vi "PicoLog_DATA.vi"(3 "sampleInterval_ms":dbl, 4 "handle":i16, 5 "noOfChannels":i16) -> (0 "Sensor3":i32[](graph), 1 "Waveform Graph 3":dynamicdata(graph), 2 "handle":i16)   [LabVIEW 2014]
uses:
  picohrdl.dll
panel:
  out "Sensor3 2":dynamicdata(graph)
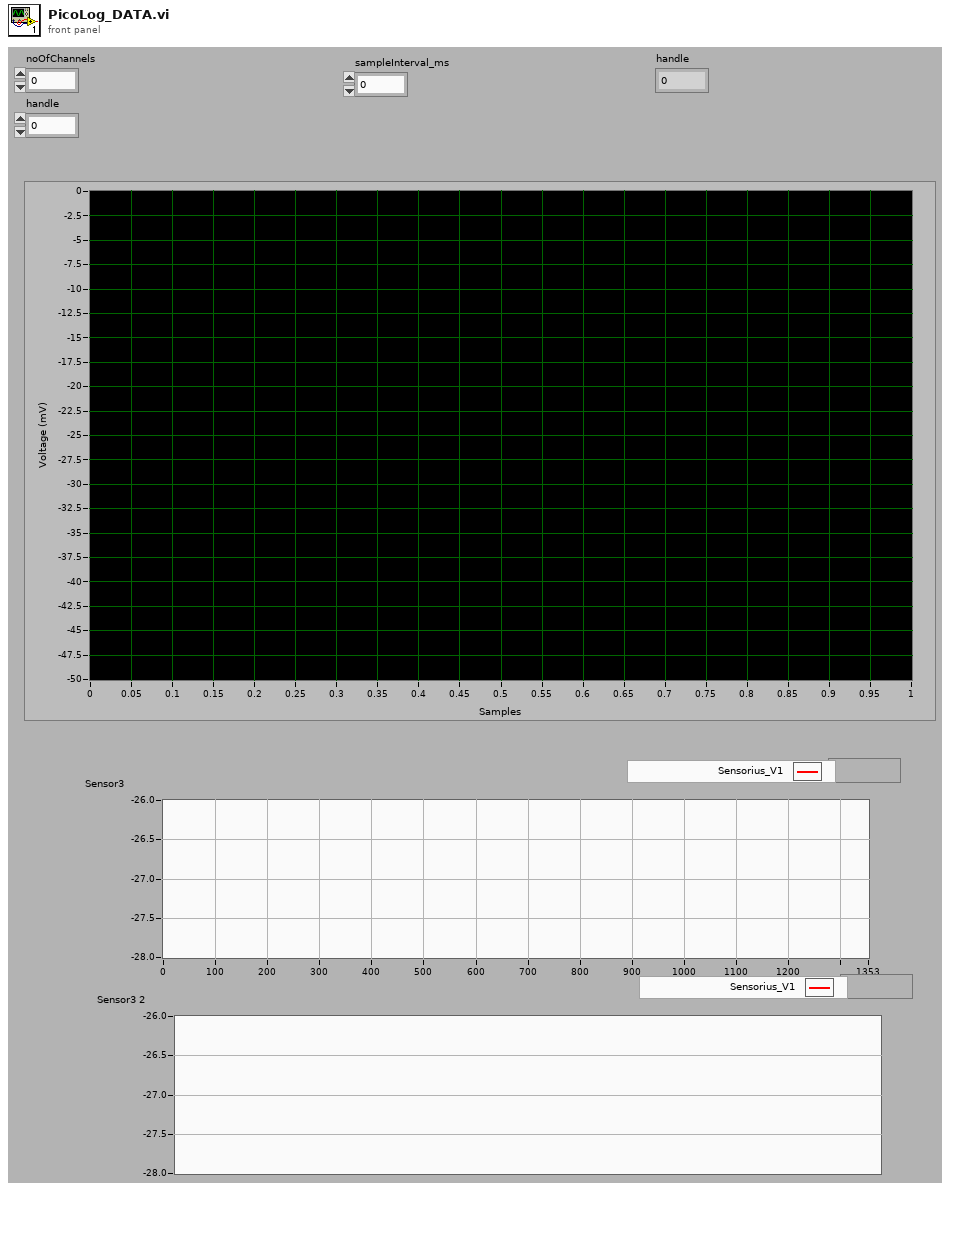
[diagram p1: front panel]
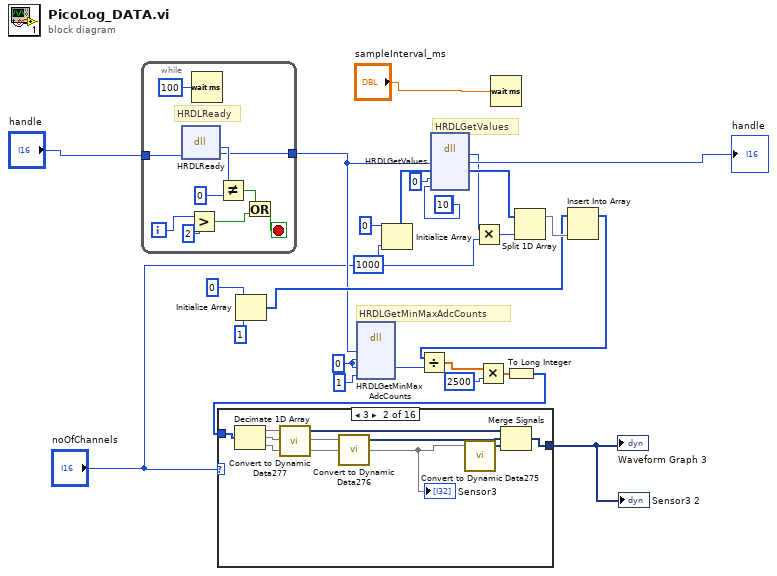
[diagram p0: block diagram]
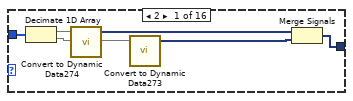
[diagram p2: hidden frame]
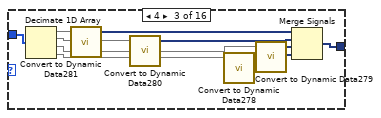
[diagram p3: hidden frame]
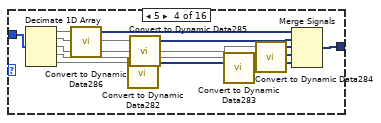
[diagram p4: hidden frame]
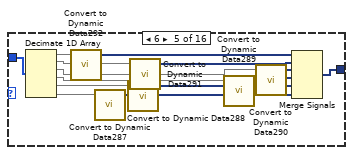
[diagram p5: hidden frame]
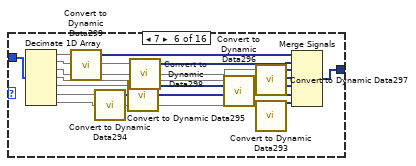
[diagram p6: hidden frame]
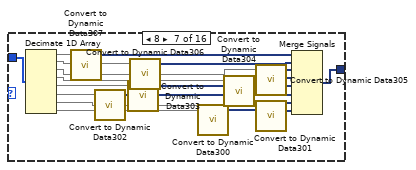
[diagram p7: hidden frame]
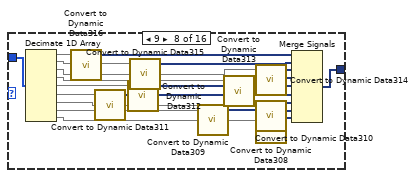
[diagram p8: hidden frame]
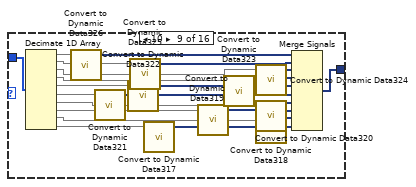
[diagram p9: hidden frame]
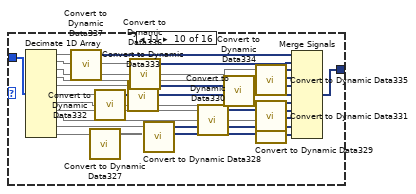
[diagram p10: hidden frame]
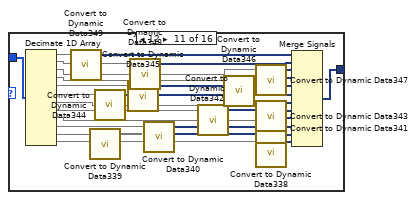
[diagram p11: hidden frame]
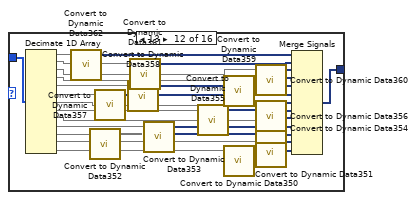
[diagram p12: hidden frame]
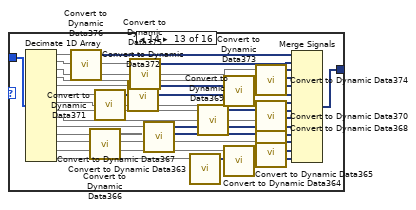
[diagram p13: hidden frame]
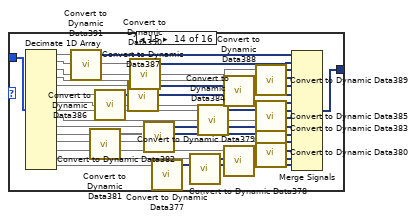
[diagram p14: hidden frame]
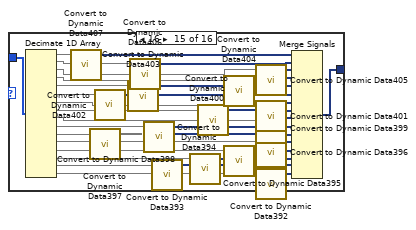
[diagram p15: hidden frame]
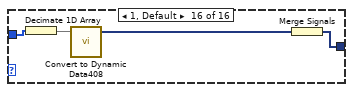
[diagram p16: hidden frame]
diagram:
  w19 = 0 ("maxAdc")
  (unwired) 10 ("noOfValues")
  # "HRDLGetMinMaxAdcCounts"
  # "HRDLGetValues"
  n1 = while {
    tunnel: "handle" -> [w34]
    tunnel: [w33] -> w3
    i -> [w31]
    stop <- w29 stop-if-true
    # "HRDLReady"
    n2 = dll-call lib="PicoHRDL.dll" fn="HRDLReady"("handle"=w34) -> ("ready"=w36:i16, "handle"=w33:i16)  [unwired: 3 in, 2 out]
    n3 = Greater?(x=w31, y=2) -> (0:w27:bool)
    n4 = Wait (ms)(milliseconds to wait=u32 100) -> ()  [unwired: 1 out]
    n5 = Not Equal?(x=w36, y=i16 0) -> (x != y?=w28:bool)
    n6 = Or(x=w28, y=w27) -> (x .or. y?=w29:bool)
  }
  n7 = Initialize Array(0 ("element"), 1 ("dimension size")) -> (w5:i32[])
  n8 = dll-call lib="PicoHRDL.dll" fn="HRDLGetMinMaxAdcCounts"("handle"=w3, "minAdc"=w19, "maxAdc"=w19, "channel"=i16 1) -> ("maxAdc"=w9:i32)  [unwired: 7 in, 2 out]
  n9 = Initialize Array(0 ("element"), 1000 ("dimension size")) -> (w26:i32[])
  n10 = dll-call lib="PicoHRDL.dll" fn="HRDLGetValues"("handle"=w3, "values"=w26, "overflow"=i16 0, "noOfValues"=10) -> ("noValuesPerChan"=w12:i32, "handle"=→"handle":i16, "values"=w14:i32[])  [unwired: 5 in, 2 out]
  n11 = Multiply(x=w12, y="noOfChannels") -> (x*y=w13:i32)
  n12 = Wait (ms)(milliseconds to wait="sampleInterval_ms") -> ()  [unwired: 1 out]
  n13 = Split 1D Array(array=w14, index=w13) -> (first subarray=w11:i32[])  [unwired: 1 out]
  n14 = Insert Into Array(array=w5, new element=w11) -> (w15:i32[])  [unwired: 1 in]
  n15 = Divide(x=w15, y=w9) -> (x/y=w18:dbl[])
  n16 = Multiply(x=w18, y=2500 ("noOfValues")) -> (x*y=w17:dbl[])
  n17 = To Long Integer(number=w17) -> (32bit integer=w10:i32[])
  n18 = case shown="3" "noOfChannels" {
    tunnel: [w38 w46 w56 w68 w82 w98 w116 w136 w158 w182 w208 w236 w266 w298 w332 w338] -> w1
    tunnel: w10 -> [w37 w45 w55 w67 w81 w97 w115 w135 w157 w181 w207 w235 w265 w297 w331 w337]
    frame 2 {
      n19 = Decimate 1D Array(w37) -> (w39:i32[], w41:i32[])
      n20 = call "Convert to Dynamic Data274"("Array"=w39) -> ("Dynamic Data Type"=w40:dynamicdata)  [unwired: 3 in]
      n21 = call "Convert to Dynamic Data273"("Array"=w41) -> ("Dynamic Data Type"=w42:dynamicdata)  [unwired: 3 in]
      n22 = Merge Signals(w40, w42) -> (w38:dynamicdata)
    }
    frame 3 {
      n23 = Decimate 1D Array(w45) -> (w47:i32[], w49:i32[], w43:i32[])
      "Sensor3" <- w43
      n24 = call "Convert to Dynamic Data277"("Array"=w47) -> ("Dynamic Data Type"=w48:dynamicdata)  [unwired: 3 in]
      n25 = call "Convert to Dynamic Data276"("Array"=w49) -> ("Dynamic Data Type"=w50:dynamicdata)  [unwired: 3 in]
      n26 = call "Convert to Dynamic Data275"("Array"=w43) -> ("Dynamic Data Type"=w44:dynamicdata)  [unwired: 3 in]
      n27 = Merge Signals(w48, w50, w44) -> (w46:dynamicdata)
    }
    frame 4 {
      n28 = Decimate 1D Array(w55) -> (w57:i32[], w59:i32[], w54:i32[], w52:i32[])
      n29 = call "Convert to Dynamic Data281"("Array"=w57) -> ("Dynamic Data Type"=w58:dynamicdata)  [unwired: 3 in]
      n30 = call "Convert to Dynamic Data280"("Array"=w59) -> ("Dynamic Data Type"=w60:dynamicdata)  [unwired: 3 in]
      n31 = call "Convert to Dynamic Data278"("Array"=w52) -> ("Dynamic Data Type"=w51:dynamicdata)  [unwired: 3 in]
      n32 = call "Convert to Dynamic Data279"("Array"=w54) -> ("Dynamic Data Type"=w53:dynamicdata)  [unwired: 3 in]
      n33 = Merge Signals(w58, w60, w53, w51) -> (w56:dynamicdata)
    }
    frame 5 {
      n34 = Decimate 1D Array(w67) -> (w69:i32[], w71:i32[], w66:i32[], w64:i32[], w62:i32[])
      n35 = call "Convert to Dynamic Data286"("Array"=w69) -> ("Dynamic Data Type"=w70:dynamicdata)  [unwired: 3 in]
      n36 = call "Convert to Dynamic Data282"("Array"=w62) -> ("Dynamic Data Type"=w61:dynamicdata)  [unwired: 3 in]
      n37 = call "Convert to Dynamic Data285"("Array"=w71) -> ("Dynamic Data Type"=w72:dynamicdata)  [unwired: 3 in]
      n38 = call "Convert to Dynamic Data283"("Array"=w64) -> ("Dynamic Data Type"=w63:dynamicdata)  [unwired: 3 in]
      n39 = call "Convert to Dynamic Data284"("Array"=w66) -> ("Dynamic Data Type"=w65:dynamicdata)  [unwired: 3 in]
      n40 = Merge Signals(w70, w72, w65, w63, w61) -> (w68:dynamicdata)
    }
    frame 6 {
      n41 = Decimate 1D Array(w81) -> (w83:i32[], w85:i32[], w80:i32[], w78:i32[], w76:i32[], w74:i32[])
      n42 = call "Convert to Dynamic Data292"("Array"=w83) -> ("Dynamic Data Type"=w84:dynamicdata)  [unwired: 3 in]
      n43 = call "Convert to Dynamic Data287"("Array"=w74) -> ("Dynamic Data Type"=w73:dynamicdata)  [unwired: 3 in]
      n44 = call "Convert to Dynamic Data288"("Array"=w76) -> ("Dynamic Data Type"=w75:dynamicdata)  [unwired: 3 in]
      n45 = call "Convert to Dynamic Data291"("Array"=w85) -> ("Dynamic Data Type"=w86:dynamicdata)  [unwired: 3 in]
      n46 = call "Convert to Dynamic Data289"("Array"=w78) -> ("Dynamic Data Type"=w77:dynamicdata)  [unwired: 3 in]
      n47 = call "Convert to Dynamic Data290"("Array"=w80) -> ("Dynamic Data Type"=w79:dynamicdata)  [unwired: 3 in]
      n48 = Merge Signals(w84, w86, w79, w77, w75, w73) -> (w82:dynamicdata)
    }
    frame 7 {
      n49 = Decimate 1D Array(w97) -> (w99:i32[], w101:i32[], w96:i32[], w94:i32[], w92:i32[], w90:i32[], w88:i32[])
      n50 = call "Convert to Dynamic Data299"("Array"=w99) -> ("Dynamic Data Type"=w100:dynamicdata)  [unwired: 3 in]
      n51 = call "Convert to Dynamic Data294"("Array"=w90) -> ("Dynamic Data Type"=w89:dynamicdata)  [unwired: 3 in]
      n52 = call "Convert to Dynamic Data295"("Array"=w92) -> ("Dynamic Data Type"=w91:dynamicdata)  [unwired: 3 in]
      n53 = call "Convert to Dynamic Data298"("Array"=w101) -> ("Dynamic Data Type"=w102:dynamicdata)  [unwired: 3 in]
      n54 = call "Convert to Dynamic Data296"("Array"=w94) -> ("Dynamic Data Type"=w93:dynamicdata)  [unwired: 3 in]
      n55 = call "Convert to Dynamic Data297"("Array"=w96) -> ("Dynamic Data Type"=w95:dynamicdata)  [unwired: 3 in]
      n56 = call "Convert to Dynamic Data293"("Array"=w88) -> ("Dynamic Data Type"=w87:dynamicdata)  [unwired: 3 in]
      n57 = Merge Signals(w100, w102, w95, w93, w91, w89, w87) -> (w98:dynamicdata)
    }
    frame 8 {
      n58 = Decimate 1D Array(w115) -> (w117:i32[], w119:i32[], w114:i32[], w112:i32[], w110:i32[], w108:i32[], w106:i32[], w104:i32[])
      n59 = call "Convert to Dynamic Data307"("Array"=w117) -> ("Dynamic Data Type"=w118:dynamicdata)  [unwired: 3 in]
      n60 = call "Convert to Dynamic Data302"("Array"=w108) -> ("Dynamic Data Type"=w107:dynamicdata)  [unwired: 3 in]
      n61 = call "Convert to Dynamic Data303"("Array"=w110) -> ("Dynamic Data Type"=w109:dynamicdata)  [unwired: 3 in]
      n62 = call "Convert to Dynamic Data306"("Array"=w119) -> ("Dynamic Data Type"=w120:dynamicdata)  [unwired: 3 in]
      n63 = call "Convert to Dynamic Data300"("Array"=w104) -> ("Dynamic Data Type"=w103:dynamicdata)  [unwired: 3 in]
      n64 = call "Convert to Dynamic Data304"("Array"=w112) -> ("Dynamic Data Type"=w111:dynamicdata)  [unwired: 3 in]
      n65 = call "Convert to Dynamic Data305"("Array"=w114) -> ("Dynamic Data Type"=w113:dynamicdata)  [unwired: 3 in]
      n66 = call "Convert to Dynamic Data301"("Array"=w106) -> ("Dynamic Data Type"=w105:dynamicdata)  [unwired: 3 in]
      n67 = Merge Signals(w118, w120, w113, w111, w109, w107, w105, w103) -> (w116:dynamicdata)
    }
    frame 9 {
      n68 = Decimate 1D Array(w135) -> (w137:i32[], w139:i32[], w134:i32[], w132:i32[], w130:i32[], w128:i32[], w126:i32[], w124:i32[], w122:i32[])
      n69 = call "Convert to Dynamic Data316"("Array"=w137) -> ("Dynamic Data Type"=w138:dynamicdata)  [unwired: 3 in]
      n70 = call "Convert to Dynamic Data311"("Array"=w128) -> ("Dynamic Data Type"=w127:dynamicdata)  [unwired: 3 in]
      n71 = call "Convert to Dynamic Data312"("Array"=w130) -> ("Dynamic Data Type"=w129:dynamicdata)  [unwired: 3 in]
      n72 = call "Convert to Dynamic Data315"("Array"=w139) -> ("Dynamic Data Type"=w140:dynamicdata)  [unwired: 3 in]
      n73 = call "Convert to Dynamic Data309"("Array"=w124) -> ("Dynamic Data Type"=w123:dynamicdata)  [unwired: 3 in]
      n74 = call "Convert to Dynamic Data313"("Array"=w132) -> ("Dynamic Data Type"=w131:dynamicdata)  [unwired: 3 in]
      n75 = call "Convert to Dynamic Data314"("Array"=w134) -> ("Dynamic Data Type"=w133:dynamicdata)  [unwired: 3 in]
      n76 = call "Convert to Dynamic Data310"("Array"=w126) -> ("Dynamic Data Type"=w125:dynamicdata)  [unwired: 3 in]
      n77 = call "Convert to Dynamic Data308"("Array"=w122) -> ("Dynamic Data Type"=w121:dynamicdata)  [unwired: 3 in]
      n78 = Merge Signals(w138, w140, w133, w131, w129, w127, w125, w123, w121) -> (w136:dynamicdata)
    }
    frame 10 {
      n79 = Decimate 1D Array(w157) -> (w159:i32[], w161:i32[], w156:i32[], w154:i32[], w152:i32[], w150:i32[], w148:i32[], w146:i32[], w144:i32[], w142:i32[])
      n80 = call "Convert to Dynamic Data326"("Array"=w159) -> ("Dynamic Data Type"=w160:dynamicdata)  [unwired: 3 in]
      n81 = call "Convert to Dynamic Data321"("Array"=w150) -> ("Dynamic Data Type"=w149:dynamicdata)  [unwired: 3 in]
      n82 = call "Convert to Dynamic Data322"("Array"=w152) -> ("Dynamic Data Type"=w151:dynamicdata)  [unwired: 3 in]
      n83 = call "Convert to Dynamic Data325"("Array"=w161) -> ("Dynamic Data Type"=w162:dynamicdata)  [unwired: 3 in]
      n84 = call "Convert to Dynamic Data317"("Array"=w142) -> ("Dynamic Data Type"=w141:dynamicdata)  [unwired: 3 in]
      n85 = call "Convert to Dynamic Data319"("Array"=w146) -> ("Dynamic Data Type"=w145:dynamicdata)  [unwired: 3 in]
      n86 = call "Convert to Dynamic Data323"("Array"=w154) -> ("Dynamic Data Type"=w153:dynamicdata)  [unwired: 3 in]
      n87 = call "Convert to Dynamic Data324"("Array"=w156) -> ("Dynamic Data Type"=w155:dynamicdata)  [unwired: 3 in]
      n88 = call "Convert to Dynamic Data320"("Array"=w148) -> ("Dynamic Data Type"=w147:dynamicdata)  [unwired: 3 in]
      n89 = call "Convert to Dynamic Data318"("Array"=w144) -> ("Dynamic Data Type"=w143:dynamicdata)  [unwired: 3 in]
      n90 = Merge Signals(w160, w162, w155, w153, w151, w149, w147, w145, w143, w141) -> (w158:dynamicdata)
    }
    frame 11 {
      n91 = Decimate 1D Array(w181) -> (w183:i32[], w185:i32[], w180:i32[], w178:i32[], w176:i32[], w174:i32[], w172:i32[], w170:i32[], w168:i32[], w166:i32[], w164:i32[])
      n92 = call "Convert to Dynamic Data337"("Array"=w183) -> ("Dynamic Data Type"=w184:dynamicdata)  [unwired: 3 in]
      n93 = call "Convert to Dynamic Data327"("Array"=w164) -> ("Dynamic Data Type"=w163:dynamicdata)  [unwired: 3 in]
      n94 = call "Convert to Dynamic Data332"("Array"=w174) -> ("Dynamic Data Type"=w173:dynamicdata)  [unwired: 3 in]
      n95 = call "Convert to Dynamic Data333"("Array"=w176) -> ("Dynamic Data Type"=w175:dynamicdata)  [unwired: 3 in]
      n96 = call "Convert to Dynamic Data336"("Array"=w185) -> ("Dynamic Data Type"=w186:dynamicdata)  [unwired: 3 in]
      n97 = call "Convert to Dynamic Data328"("Array"=w166) -> ("Dynamic Data Type"=w165:dynamicdata)  [unwired: 3 in]
      n98 = call "Convert to Dynamic Data330"("Array"=w170) -> ("Dynamic Data Type"=w169:dynamicdata)  [unwired: 3 in]
      n99 = call "Convert to Dynamic Data334"("Array"=w178) -> ("Dynamic Data Type"=w177:dynamicdata)  [unwired: 3 in]
      n100 = call "Convert to Dynamic Data335"("Array"=w180) -> ("Dynamic Data Type"=w179:dynamicdata)  [unwired: 3 in]
      n101 = call "Convert to Dynamic Data331"("Array"=w172) -> ("Dynamic Data Type"=w171:dynamicdata)  [unwired: 3 in]
      n102 = call "Convert to Dynamic Data329"("Array"=w168) -> ("Dynamic Data Type"=w167:dynamicdata)  [unwired: 3 in]
      n103 = Merge Signals(w184, w186, w179, w177, w175, w173, w171, w169, w167, w165, w163) -> (w182:dynamicdata)
    }
    frame 12 {
      n104 = Decimate 1D Array(w207) -> (w209:i32[], w211:i32[], w206:i32[], w204:i32[], w202:i32[], w200:i32[], w198:i32[], w196:i32[], w194:i32[], w192:i32[], w190:i32[], w188:i32[])
      n105 = call "Convert to Dynamic Data349"("Array"=w209) -> ("Dynamic Data Type"=w210:dynamicdata)  [unwired: 3 in]
      n106 = call "Convert to Dynamic Data339"("Array"=w190) -> ("Dynamic Data Type"=w189:dynamicdata)  [unwired: 3 in]
      n107 = call "Convert to Dynamic Data344"("Array"=w200) -> ("Dynamic Data Type"=w199:dynamicdata)  [unwired: 3 in]
      n108 = call "Convert to Dynamic Data345"("Array"=w202) -> ("Dynamic Data Type"=w201:dynamicdata)  [unwired: 3 in]
      n109 = call "Convert to Dynamic Data348"("Array"=w211) -> ("Dynamic Data Type"=w212:dynamicdata)  [unwired: 3 in]
      n110 = call "Convert to Dynamic Data340"("Array"=w192) -> ("Dynamic Data Type"=w191:dynamicdata)  [unwired: 3 in]
      n111 = call "Convert to Dynamic Data342"("Array"=w196) -> ("Dynamic Data Type"=w195:dynamicdata)  [unwired: 3 in]
      n112 = call "Convert to Dynamic Data346"("Array"=w204) -> ("Dynamic Data Type"=w203:dynamicdata)  [unwired: 3 in]
      n113 = call "Convert to Dynamic Data347"("Array"=w206) -> ("Dynamic Data Type"=w205:dynamicdata)  [unwired: 3 in]
      n114 = call "Convert to Dynamic Data343"("Array"=w198) -> ("Dynamic Data Type"=w197:dynamicdata)  [unwired: 3 in]
      n115 = call "Convert to Dynamic Data341"("Array"=w194) -> ("Dynamic Data Type"=w193:dynamicdata)  [unwired: 3 in]
      n116 = call "Convert to Dynamic Data338"("Array"=w188) -> ("Dynamic Data Type"=w187:dynamicdata)  [unwired: 3 in]
      n117 = Merge Signals(w210, w212, w205, w203, w201, w199, w197, w195, w193, w191, w189, w187) -> (w208:dynamicdata)
    }
    frame 13 {
      n118 = Decimate 1D Array(w235) -> (w237:i32[], w239:i32[], w234:i32[], w232:i32[], w230:i32[], w228:i32[], w226:i32[], w224:i32[], w222:i32[], w220:i32[], w218:i32[], w216:i32[], w214:i32[])
      n119 = call "Convert to Dynamic Data362"("Array"=w237) -> ("Dynamic Data Type"=w238:dynamicdata)  [unwired: 3 in]
      n120 = call "Convert to Dynamic Data352"("Array"=w218) -> ("Dynamic Data Type"=w217:dynamicdata)  [unwired: 3 in]
      n121 = call "Convert to Dynamic Data357"("Array"=w228) -> ("Dynamic Data Type"=w227:dynamicdata)  [unwired: 3 in]
      n122 = call "Convert to Dynamic Data358"("Array"=w230) -> ("Dynamic Data Type"=w229:dynamicdata)  [unwired: 3 in]
      n123 = call "Convert to Dynamic Data361"("Array"=w239) -> ("Dynamic Data Type"=w240:dynamicdata)  [unwired: 3 in]
      n124 = call "Convert to Dynamic Data353"("Array"=w220) -> ("Dynamic Data Type"=w219:dynamicdata)  [unwired: 3 in]
      n125 = call "Convert to Dynamic Data355"("Array"=w224) -> ("Dynamic Data Type"=w223:dynamicdata)  [unwired: 3 in]
      n126 = call "Convert to Dynamic Data359"("Array"=w232) -> ("Dynamic Data Type"=w231:dynamicdata)  [unwired: 3 in]
      n127 = call "Convert to Dynamic Data350"("Array"=w214) -> ("Dynamic Data Type"=w213:dynamicdata)  [unwired: 3 in]
      n128 = call "Convert to Dynamic Data360"("Array"=w234) -> ("Dynamic Data Type"=w233:dynamicdata)  [unwired: 3 in]
      n129 = call "Convert to Dynamic Data356"("Array"=w226) -> ("Dynamic Data Type"=w225:dynamicdata)  [unwired: 3 in]
      n130 = call "Convert to Dynamic Data354"("Array"=w222) -> ("Dynamic Data Type"=w221:dynamicdata)  [unwired: 3 in]
      n131 = call "Convert to Dynamic Data351"("Array"=w216) -> ("Dynamic Data Type"=w215:dynamicdata)  [unwired: 3 in]
      n132 = Merge Signals(w238, w240, w233, w231, w229, w227, w225, w223, w221, w219, w217, w215, w213) -> (w236:dynamicdata)
    }
    frame 14 {
      n133 = Decimate 1D Array(w265) -> (w267:i32[], w269:i32[], w264:i32[], w262:i32[], w260:i32[], w258:i32[], w256:i32[], w254:i32[], w252:i32[], w250:i32[], w248:i32[], w246:i32[], w244:i32[], w242:i32[])
      n134 = call "Convert to Dynamic Data376"("Array"=w267) -> ("Dynamic Data Type"=w268:dynamicdata)  [unwired: 3 in]
      n135 = call "Convert to Dynamic Data366"("Array"=w248) -> ("Dynamic Data Type"=w247:dynamicdata)  [unwired: 3 in]
      n136 = call "Convert to Dynamic Data371"("Array"=w258) -> ("Dynamic Data Type"=w257:dynamicdata)  [unwired: 3 in]
      n137 = call "Convert to Dynamic Data372"("Array"=w260) -> ("Dynamic Data Type"=w259:dynamicdata)  [unwired: 3 in]
      n138 = call "Convert to Dynamic Data375"("Array"=w269) -> ("Dynamic Data Type"=w270:dynamicdata)  [unwired: 3 in]
      n139 = call "Convert to Dynamic Data367"("Array"=w250) -> ("Dynamic Data Type"=w249:dynamicdata)  [unwired: 3 in]
      n140 = call "Convert to Dynamic Data363"("Array"=w242) -> ("Dynamic Data Type"=w241:dynamicdata)  [unwired: 3 in]
      n141 = call "Convert to Dynamic Data369"("Array"=w254) -> ("Dynamic Data Type"=w253:dynamicdata)  [unwired: 3 in]
      n142 = call "Convert to Dynamic Data373"("Array"=w262) -> ("Dynamic Data Type"=w261:dynamicdata)  [unwired: 3 in]
      n143 = call "Convert to Dynamic Data364"("Array"=w244) -> ("Dynamic Data Type"=w243:dynamicdata)  [unwired: 3 in]
      n144 = call "Convert to Dynamic Data374"("Array"=w264) -> ("Dynamic Data Type"=w263:dynamicdata)  [unwired: 3 in]
      n145 = call "Convert to Dynamic Data370"("Array"=w256) -> ("Dynamic Data Type"=w255:dynamicdata)  [unwired: 3 in]
      n146 = call "Convert to Dynamic Data368"("Array"=w252) -> ("Dynamic Data Type"=w251:dynamicdata)  [unwired: 3 in]
      n147 = call "Convert to Dynamic Data365"("Array"=w246) -> ("Dynamic Data Type"=w245:dynamicdata)  [unwired: 3 in]
      n148 = Merge Signals(w268, w270, w263, w261, w259, w257, w255, w253, w251, w249, w247, w245, w243, w241) -> (w266:dynamicdata)
    }
    frame 15 {
      n149 = Decimate 1D Array(w297) -> (w299:i32[], w301:i32[], w296:i32[], w294:i32[], w292:i32[], w290:i32[], w288:i32[], w286:i32[], w284:i32[], w282:i32[], w280:i32[], w278:i32[], w276:i32[], w274:i32[], w272:i32[])
      n150 = call "Convert to Dynamic Data391"("Array"=w299) -> ("Dynamic Data Type"=w300:dynamicdata)  [unwired: 3 in]
      n151 = call "Convert to Dynamic Data381"("Array"=w280) -> ("Dynamic Data Type"=w279:dynamicdata)  [unwired: 3 in]
      n152 = call "Convert to Dynamic Data386"("Array"=w290) -> ("Dynamic Data Type"=w289:dynamicdata)  [unwired: 3 in]
      n153 = call "Convert to Dynamic Data387"("Array"=w292) -> ("Dynamic Data Type"=w291:dynamicdata)  [unwired: 3 in]
      n154 = call "Convert to Dynamic Data390"("Array"=w301) -> ("Dynamic Data Type"=w302:dynamicdata)  [unwired: 3 in]
      n155 = call "Convert to Dynamic Data382"("Array"=w282) -> ("Dynamic Data Type"=w281:dynamicdata)  [unwired: 3 in]
      n156 = call "Convert to Dynamic Data377"("Array"=w272) -> ("Dynamic Data Type"=w271:dynamicdata)  [unwired: 3 in]
      n157 = call "Convert to Dynamic Data378"("Array"=w274) -> ("Dynamic Data Type"=w273:dynamicdata)  [unwired: 3 in]
      n158 = call "Convert to Dynamic Data384"("Array"=w286) -> ("Dynamic Data Type"=w285:dynamicdata)  [unwired: 3 in]
      n159 = call "Convert to Dynamic Data388"("Array"=w294) -> ("Dynamic Data Type"=w293:dynamicdata)  [unwired: 3 in]
      n160 = call "Convert to Dynamic Data379"("Array"=w276) -> ("Dynamic Data Type"=w275:dynamicdata)  [unwired: 3 in]
      n161 = call "Convert to Dynamic Data389"("Array"=w296) -> ("Dynamic Data Type"=w295:dynamicdata)  [unwired: 3 in]
      n162 = call "Convert to Dynamic Data385"("Array"=w288) -> ("Dynamic Data Type"=w287:dynamicdata)  [unwired: 3 in]
      n163 = call "Convert to Dynamic Data383"("Array"=w284) -> ("Dynamic Data Type"=w283:dynamicdata)  [unwired: 3 in]
      n164 = call "Convert to Dynamic Data380"("Array"=w278) -> ("Dynamic Data Type"=w277:dynamicdata)  [unwired: 3 in]
      n165 = Merge Signals(w300, w302, w295, w293, w291, w289, w287, w285, w283, w281, w279, w277, w275, w273, w271) -> (w298:dynamicdata)
    }
    frame 16 {
      n166 = Decimate 1D Array(w331) -> (w333:i32[], w335:i32[], w330:i32[], w328:i32[], w326:i32[], w324:i32[], w322:i32[], w320:i32[], w318:i32[], w316:i32[], w314:i32[], w312:i32[], w310:i32[], w308:i32[], w306:i32[], w304:i32[])
      n167 = call "Convert to Dynamic Data407"("Array"=w333) -> ("Dynamic Data Type"=w334:dynamicdata)  [unwired: 3 in]
      n168 = call "Convert to Dynamic Data397"("Array"=w314) -> ("Dynamic Data Type"=w313:dynamicdata)  [unwired: 3 in]
      n169 = call "Convert to Dynamic Data402"("Array"=w324) -> ("Dynamic Data Type"=w323:dynamicdata)  [unwired: 3 in]
      n170 = call "Convert to Dynamic Data403"("Array"=w326) -> ("Dynamic Data Type"=w325:dynamicdata)  [unwired: 3 in]
      n171 = call "Convert to Dynamic Data406"("Array"=w335) -> ("Dynamic Data Type"=w336:dynamicdata)  [unwired: 3 in]
      n172 = call "Convert to Dynamic Data398"("Array"=w316) -> ("Dynamic Data Type"=w315:dynamicdata)  [unwired: 3 in]
      n173 = call "Convert to Dynamic Data393"("Array"=w306) -> ("Dynamic Data Type"=w305:dynamicdata)  [unwired: 3 in]
      n174 = call "Convert to Dynamic Data394"("Array"=w308) -> ("Dynamic Data Type"=w307:dynamicdata)  [unwired: 3 in]
      n175 = call "Convert to Dynamic Data400"("Array"=w320) -> ("Dynamic Data Type"=w319:dynamicdata)  [unwired: 3 in]
      n176 = call "Convert to Dynamic Data404"("Array"=w328) -> ("Dynamic Data Type"=w327:dynamicdata)  [unwired: 3 in]
      n177 = call "Convert to Dynamic Data395"("Array"=w310) -> ("Dynamic Data Type"=w309:dynamicdata)  [unwired: 3 in]
      n178 = call "Convert to Dynamic Data405"("Array"=w330) -> ("Dynamic Data Type"=w329:dynamicdata)  [unwired: 3 in]
      n179 = call "Convert to Dynamic Data401"("Array"=w322) -> ("Dynamic Data Type"=w321:dynamicdata)  [unwired: 3 in]
      n180 = call "Convert to Dynamic Data399"("Array"=w318) -> ("Dynamic Data Type"=w317:dynamicdata)  [unwired: 3 in]
      n181 = call "Convert to Dynamic Data396"("Array"=w312) -> ("Dynamic Data Type"=w311:dynamicdata)  [unwired: 3 in]
      n182 = call "Convert to Dynamic Data392"("Array"=w304) -> ("Dynamic Data Type"=w303:dynamicdata)  [unwired: 3 in]
      n183 = Merge Signals(w334, w336, w329, w327, w325, w323, w321, w319, w317, w315, w313, w311, w309, w307, w305, w303) -> (w332:dynamicdata)
    }
    frame 1, Default {
      n184 = Decimate 1D Array(w337) -> (w339:i32[])
      n185 = call "Convert to Dynamic Data408"("Array"=w339) -> ("Dynamic Data Type"=w340:dynamicdata)  [unwired: 3 in]
      n186 = Merge Signals(w340) -> (w338:dynamicdata)
    }
  }
  "Waveform Graph 3" <- w1
  "Sensor3 2" <- w1
